vi "Function_generator.vi"(0 "task in":refnum<k21>, 1 "frequency":dbl=1000.0 format="%.2f", 2 "physical channels":tag, 3 "error in":errorcluster, 4 "offset":dbl format="%.2f", 5 "amplitude":dbl=5.0 format="%.2f") -> (6 "task out":refnum<k21>, 9 "error out":errorcluster)   [LabVIEW 2023]
uses:
  <vilib>/DAQmx/create/channels.llb/DAQmx Create Channel (AO-FuncGen).vi
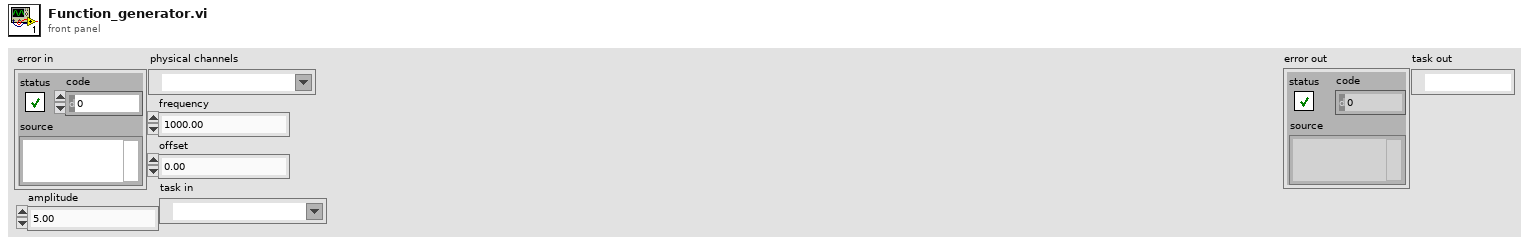
[diagram p1: front panel]
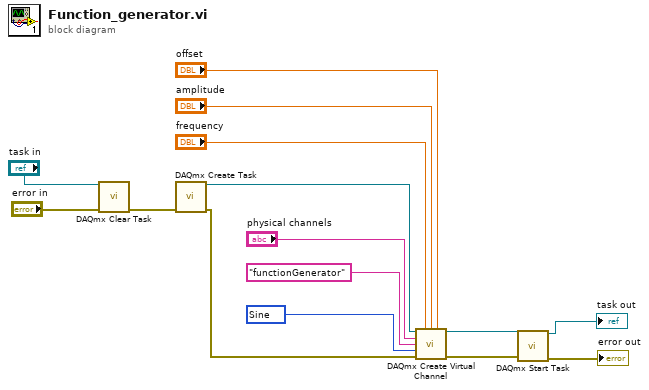
[diagram p0: block diagram]
diagram:
  w15 = 14751 items=["Sine"=14751, "Triangle"=14752, "Square"=14753, "Sawtooth"=14754] ("type")
  n1 = call <vilib>:"DAQmx Clear Task.vi"("task in"="task in", "error in"="error in") -> ("error out"=w3:errorcluster)  [unwired: 13 in]
  n2 = call <vilib>:"DAQmx Create Task.vi"("error in"=w3) -> ("task out"=w12:refnum<k21>, "error out"=w11:errorcluster)  [unwired: 13 in]
  n3 = call-poly <vilib>:"DAQmx Create Virtual Channel.vi"("task in"=w12, "frequency"="frequency", "amplitude"="amplitude", "offset"="offset", "physical channels"="physical channels", "name to assign"="functionGenerator", "type"=w15, "error in"=w11) -> ("task out"=w10:refnum<k21>, "error out"=w9:errorcluster)  [unwired: 6 in]
  n4 = call <vilib>:"DAQmx Start Task.vi"("task/channels in"=w10, "error in"=w9) -> ("task out"=→"task out":refnum<k21>, "error out"=→"error out":errorcluster)  [unwired: 12 in]
